vi "example_2_re_with_nre.vi"() -> ()   [LabVIEW 2015, in "lv_mutex_shared_1.lvlib"]
uses:
  lv_mutex_shared_1.lvlib
panel:
  in  "Wait (ms)":u32=1000
  out "Execution Time (2)":u32
  out "Execution Time (1)":u32
  out "Finish Time (2)":u32
  out "Finish Time (1)":u32
  out "Start Time":u32
  # "This VI will show that even if a VI is re-entrant, if there is a non re-entrant\nVI called within, it will still block and affect the execution time of the re-\nentrant VI."
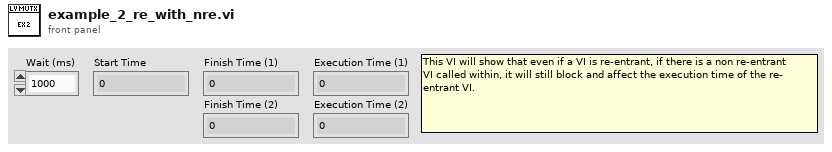
[diagram p1: front panel]
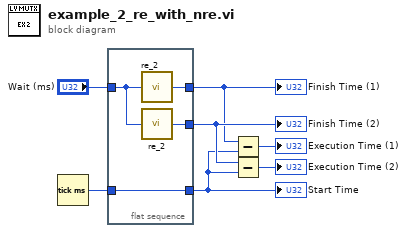
[diagram p0: block diagram]
diagram:
  n1 = Tick Count (ms)() -> (millisecond timer value=w1:u32)
  n2 = flat-sequence {
    tunnel: "Wait (ms)" -> [w11]
    tunnel: [w10] -> w4
    tunnel: [w9] -> w3
    tunnel: [w8] -> w2
    tunnel: w1 -> [w8]
    frame #0 {
      n3 = call "re_2.vi"("wait_ms"=w11) -> ("timer_ms"=w9:u32)
      n4 = call "re_2.vi"("wait_ms"=w11) -> ("timer_ms"=w10:u32)
    }
  }
  n5 = Subtract(x=w3, y=w2) -> (x-y=→"Execution Time (1)":u32)
  n6 = Subtract(x=w4, y=w2) -> (x-y=→"Execution Time (2)":u32)
  "Start Time" <- w2
  "Finish Time (1)" <- w3
  "Finish Time (2)" <- w4
